vi "Timer for auto mode.vi"(5 "Auto Profile Sequence 2":refnum<vi>, 6 "Current Sequence in":u16, 7 "ItemNames":string[][](array[string]), 8 "Total Cycle":u16, 9 "Current Cycle":u16, 10 "Write":refnum<vi>, 11 "Digital in":refnum<vi>) -> (0 "Current Cycle":u16, 1 "Test Stop":bool, 2 "Numeric":dbl, 3 "Current Sequence out":u16, 4 "number":i32)   [LabVIEW 2025]
uses:
  <vilib>/Utility/miscctls.llb/LVRowAndColumnTypeDef.ctl
  Global/Throttle.vi
panel:
  out "error out":errorcluster
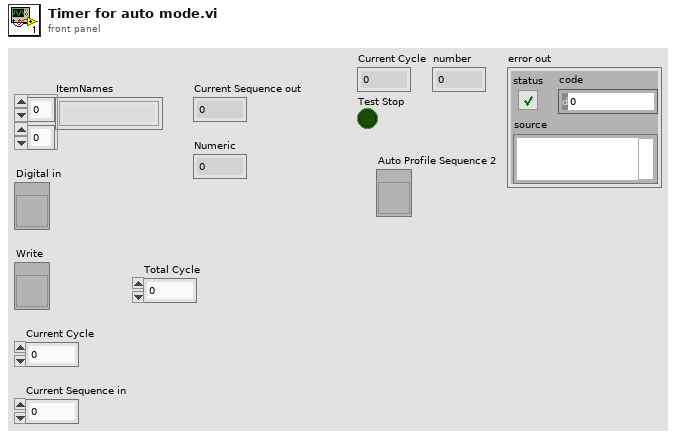
[diagram p1: front panel]
types:
  T1 = typedef "LVRowAndColumnTypeDef.ctl" = cluster{"Row":i32, "Column":i32}
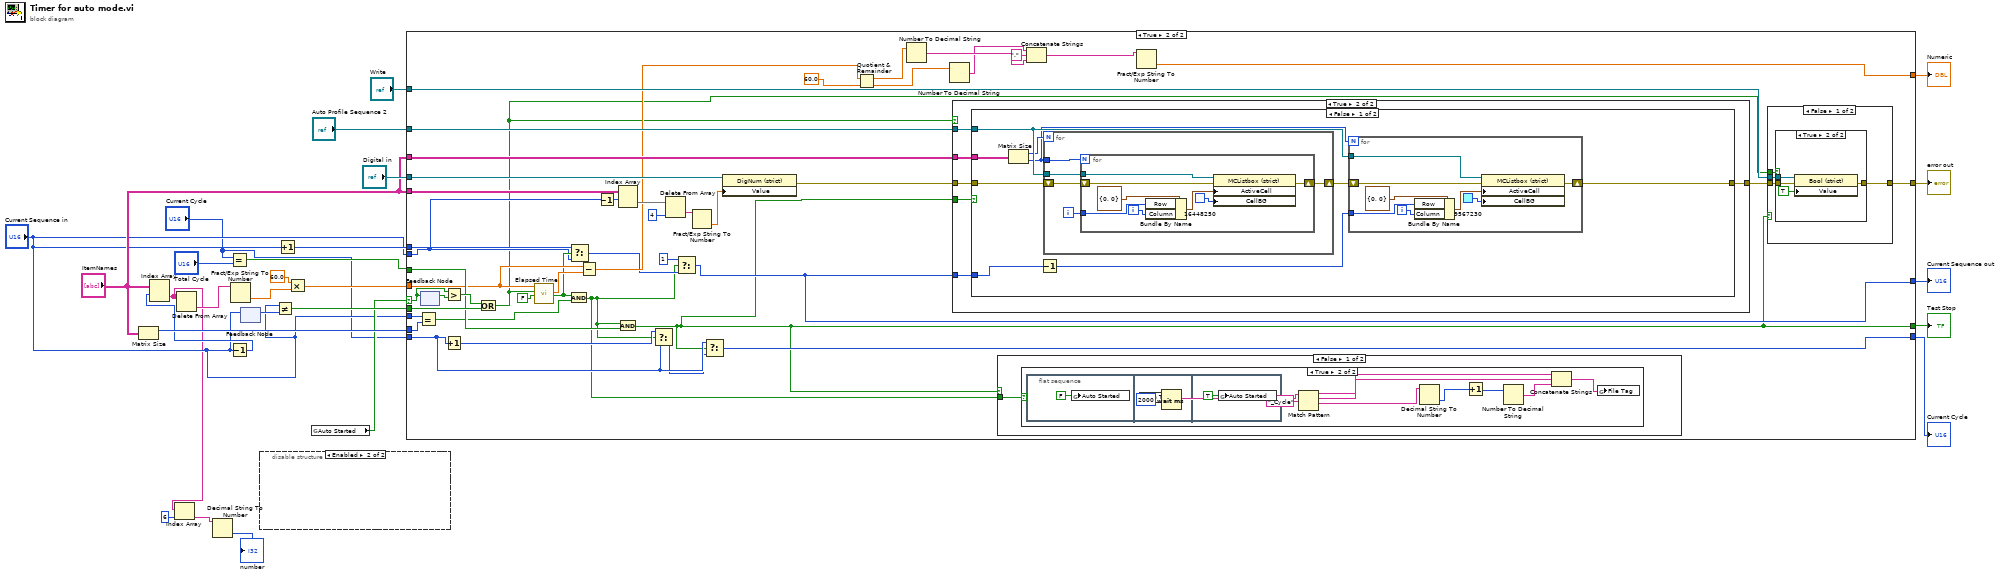
[diagram p0: block diagram]
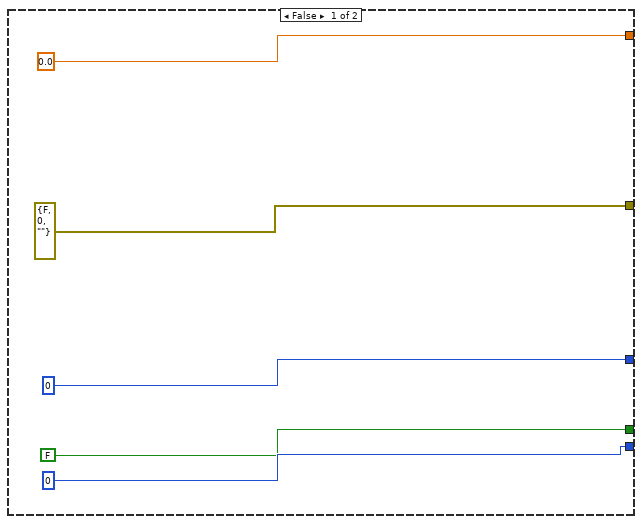
[diagram p3: hidden frame]
diagram:
  n1 = Matrix Size(0:"ItemNames") -> (1:w16:i32)  [unwired: 1 out]
  n2 = Equal?(x="Current Cycle", y="Total Cycle") -> (x = y?=w14:bool)
  n3 = Decrement(x="Current Sequence in") -> (x-1=w7:u16)
  n4 = Index Array(array="ItemNames", index (row)=w7) -> (element=w4:string[])  [unwired: 1 in]
  n5 = Index Array(array=w4, index=6) -> (element=w2:string)
  n6 = Delete From Array(array=w4) -> (deleted portion=w19:string)  [unwired: 2 in, 1 out]
  n7 = Decimal String To Number(string=w2) -> (number=→"number":i32)  [unwired: 2 in, 1 out]
  n8 = Fract/Exp String To Number(string=w19) -> (number=w20:dbl)  [unwired: 3 in, 1 out]
  n9 = feedback #1() -> (w17:u16)  [unwired: 1 in]
  n10 = feedback-in #1("Current Sequence in") -> ()
  n11 = disable-structure shown="Enabled" {
    frame Disabled {
    }
    frame Enabled {
    }
  }
  n12 = Not Equal?(x="Current Sequence in", y=w17) -> (x != y?=w18:bool)
  n13 = Increment(x="Current Sequence in") -> (x+1=w24:u16)
  n14 = Multiply(x=60.0, y=w20) -> (x*y=w21:dbl)
  n15 = global read "Throttle.vi" "Auto Started"() -> (w8:bool)
  n16 = case shown="True" w8 {
    selector: w8 -> [_ w77]
    tunnel: w18 -> [_ w75]
    tunnel: w21 -> [_ w55]
    tunnel: [0.0 w46] -> w23
    tunnel: w24 -> [_ w73]
    tunnel: "Current Sequence in" -> [_ w36]
    tunnel: [u16 0 ("Current Sequence") w39] -> w25
    tunnel: "Write" -> [_ w72]
    tunnel: "Digital in" -> [_ w71]
    tunnel: "ItemNames" -> [_ w70]
    tunnel: w16 -> [_ w66]
    tunnel: "Current Sequence in" -> [_ w65]
    tunnel: w14 -> [_ w64]
    tunnel: "Current Cycle" -> [_ w43]
    tunnel: [u16 0 ("Current Cycle") w41] -> w13
    tunnel: [FALSE w33] -> w12
    tunnel: [errorcluster {"status"=FALSE, "code"=0, "source"=""} ("error out") w63] -> w11
    tunnel: "Auto Profile Sequence 2" -> [_ w61]
    tunnel: "ItemNames" -> [_ w60]
    frame False {
    }
    frame True {
      n17 = Equal?(x=w65, y=w66) -> (x = y?=w53:bool)
      n18 = feedback-in #2(w77) -> ()
      n19 = feedback #2() -> (w78:bool)  [unwired: 1 in]
      n20 = Greater?(x=w77, y=w78) -> (0:w76:bool)
      n21 = Increment(x=w43) -> (x+1=w57:u16)
      n22 = Or(x=w76, y=w75) -> (x .or. y?=w35:bool)
      n23 = call "Elapsed Time"("Time Target (s)"=w55, "Reset"=w35, "Auto Reset"=FALSE) -> ("Elapsed Time (s)"=w54:dbl, "Time has Elapsed"=w37:bool)  [unwired: 9 in, 6 out]
      n24 = And(x=w37, y=w53) -> (x .and. y?=w34:bool)
      n25 = Select(t=w73, s=w37, f=w36) -> (s? t:f=w40:u16)
      n26 = Subtract(x=w55, y=w54) -> (x-y=w52:dbl)
      n27 = Decrement(x=w36) -> (x-1=w56:u16)
      n28 = Index Array(array=w70, index (row)=w56) -> (element=w67:string[])  [unwired: 1 in]
      n29 = And(x=w34, y=w64) -> (x .and. y?=w33:bool)
      n30 = Select(t=w57, s=w34, f=w43) -> (s? t:f=w42:u16)
      n31 = Delete From Array(array=w67, index=4) -> (deleted portion=w69:string)  [unwired: 1 in, 1 out]
      n32 = Select(t=u16 1, s=w34, f=w40) -> (s? t:f=w39:u16)
      n33 = Fract/Exp String To Number(string=w69) -> (number=w68:dbl)  [unwired: 3 in, 1 out]
      n34 = Select(t=w43, s=w33, f=w42) -> (s? t:f=w41:u16)
      n35 = property class="DigNum (strict)"(reference=w71, "Value"=w68) -> (error out=w59:errorcluster)  [unwired: 1 in, 1 out]
      n36 = Quotient & Remainder(x=w52, y=60.0) -> (x-y*floor(x/y)=w50:dbl, floor(x/y)=w49:dbl)
      n37 = Number To Decimal String(number=w50) -> (decimal integer string=w45:string)  [unwired: 1 in]
      n38 = Number To Decimal String(number=w49) -> (decimal integer string=w44:string)  [unwired: 1 in]
      n39 = case shown="True" w35 {
        tunnel: w61 -> [_ w108]
        tunnel: w60 -> [_ w107]
        tunnel: w39 -> [_ w106]
        tunnel: w59 -> [w102 w105]
        tunnel: [w102 w104] -> w58
        tunnel: w33 -> [_ w103]
        frame False {
        }
        frame True {
          n40 = case shown="False" w103 {
            tunnel: w108 -> [w117 _]
            tunnel: w107 -> [w116 _]
            tunnel: w106 -> [w115 _]
            tunnel: w105 -> [w114 w139]
            tunnel: [w113 w139] -> w104
            frame False {
              n41 = Matrix Size(0:w116) -> (1:w112:i32, 2:w110:i32)
              n42 = Decrement(x=w115) -> (x-1=w109:u16)
              n43 = for {
                N: w112 -> [_]
                tunnel: w110 -> [w130]
                shift-right: [w127] -> w111
                shift-left: w114 -> [w129]
                tunnel: w117 -> [w126]
                i -> [w128]
                n44 = for {
                  N: w130 -> [_]
                  shift-right: [w132] -> w127
                  shift-left: w129 -> [w138]
                  tunnel: w128 -> [w136]
                  tunnel: w126 -> [w131]
                  i -> [w135]
                  n45 = Bundle By Name(cluster=T1 {"Row"=0, "Column"=0} ("Active Cell:Active Cell"), "Row"=w136, "Column"=w135) -> (w134:T1)
                  n46 = property on="Property Node" class="MCListbox (strict)"(reference=w131, error in=w138, "ActiveCell"=w134, "CellBG"=u32 16448250) -> (error out=w132:errorcluster)  [unwired: 1 out]
                }
              }
              n47 = for {
                N: w110 -> [_]
                shift-right: [w119] -> w113
                shift-left: w111 -> [w125]
                tunnel: w109 -> [w123]
                tunnel: w117 -> [w118]
                i -> [w122]
                n48 = Bundle By Name(cluster=T1 {"Row"=0, "Column"=0} ("Active Cell:Active Cell"), "Row"=w123, "Column"=w122) -> (w121:T1)
                n49 = property on="Property Node" class="MCListbox (strict)"(reference=w118, error in=w125, "ActiveCell"=w121, "CellBG"=u32 9567230) -> (error out=w119:errorcluster)  [unwired: 1 out]
              }
            }
            frame True {
            }
          }
        }
      }
      n50 = case shown="False" w33 {
        tunnel: w34 -> [w79 _]
        frame False {
          n51 = case shown="True" w79 {
            frame False {
            }
            frame True {
              n52 = flat-sequence {
                frame #0 {
                  n53 = global write "Throttle.vi" "Auto Started"(FALSE ("Auto Started")) -> ()
                }
                frame #1 {
                  n54 = Wait (ms)(milliseconds to wait=u32 2000) -> ()  [unwired: 1 out]
                }
                frame #2 {
                  n55 = global write "Throttle.vi" "Auto Started"(TRUE ("Auto Started")) -> ()
                }
              }
              n56 = global read "Throttle.vi" "File Tag"() -> (w82:string)
              n57 = Match Pattern(string=w82, regular expression="_Cycle") -> (before substring=w83:string, match substring=w84:string, after substring=w85:string)  [unwired: 1 in, 1 out]
              n58 = Decimal String To Number(string=w85) -> (number=w86:i32)  [unwired: 2 in, 1 out]
              n59 = Increment(x=w86) -> (x+1=w87:i32)
              n60 = Number To Decimal String(number=w87) -> (decimal integer string=w80:string)  [unwired: 1 in]
              n61 = Concatenate Strings(w83, w84, w80) -> (w88:string)
              n62 = global write "Throttle.vi" "File Tag"(w88) -> ()
            }
          }
        }
        frame True {
        }
      }
      n63 = Concatenate Strings(w44, "." ("string"), w45) -> (w47:string)
      n64 = Fract/Exp String To Number(string=w47) -> (number=w46:dbl)  [unwired: 3 in, 1 out]
      n65 = case shown="False" w33 {
        tunnel: w72 -> [w95 _]
        tunnel: [w94 w101] -> w63
        tunnel: w58 -> [w93 w101]
        tunnel: w35 -> [w92 _]
        frame False {
          n66 = case shown="True" w92 {
            tunnel: w95 -> [_ w100]
            tunnel: [w96 w99] -> w94
            tunnel: w93 -> [w96 w98]
            frame False {
            }
            frame True {
              n67 = property class="Bool (strict)"(reference=w100, error in=w98, "Value"=TRUE) -> (error out=w99:errorcluster)  [unwired: 1 out]
            }
          }
        }
        frame True {
        }
      }
    }
  }
  "Current Sequence out" <- w25
  "Numeric" <- w23
  "Current Cycle" <- w13
  "Test Stop" <- w12
  "error out" <- w11
